vi "Encoder End.vi"(8 "error in (no error)":errorcluster, 11 "Task Out":T1) -> (0 "error out":errorcluster)   [LabVIEW 2019]
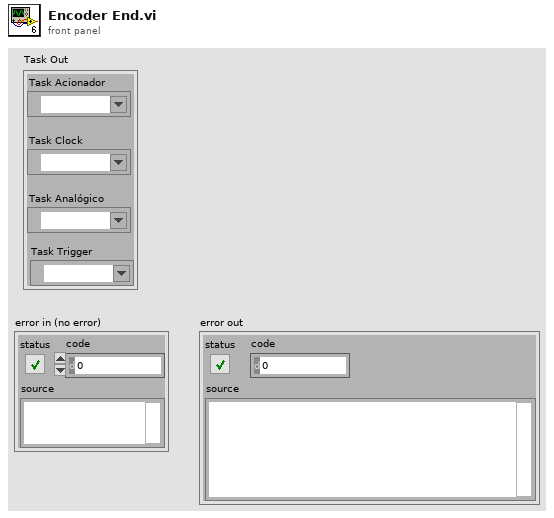
[diagram p1: front panel]
types:
  T1 = cluster{"Task Analógico":refnum<k21>, "Task Clock":refnum<k21>, "Task Acionador":refnum<k21>, "Task Trigger":tag}
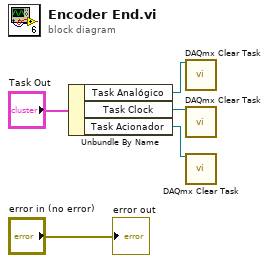
[diagram p0: block diagram]
diagram:
  n1 = Unbundle By Name("Task Out") -> ("Task Analógico"=w3:refnum<k21>, "Task Clock"=w2:refnum<k21>, "Task Acionador"=w1:refnum<k21>)
  n2 = call <vilib>:"DAQmx Clear Task.vi"("task in"=w3) -> ()  [unwired: 14 in, 1 out]
  n3 = call <vilib>:"DAQmx Clear Task.vi"("task in"=w2) -> ()  [unwired: 14 in, 1 out]
  n4 = call <vilib>:"DAQmx Clear Task.vi"("task in"=w1) -> ()  [unwired: 14 in, 1 out]
  "error out" <- "error in (no error)"
